vi "Invert Channel.vi"(8 "error in (no error)":errorcluster, 9 "Invert Channel (T: Enabled)":bool=TRUE, 10 "Channel (1: Channel 1)":u16(ring)=1 items=["Channel 1"=1, "Channel 2"=2, "Channel 3"=3, "Channel 4"=4], 11 "VISA resource name":refnum<visa-resource-name>) -> (0 "error out":errorcluster, 3 "VISA resource name out":refnum<visa-resource-name>)   [LabVIEW 2017, in "Tektronix TDS 200 1000 2000 Series.lvlib"]
doc: "Allows signals on all channels to be inverted."
uses:
  Tektronix TDS 200 1000 2000 Series.lvlib
panel:
  # "Enabled"
  # "Disabled"
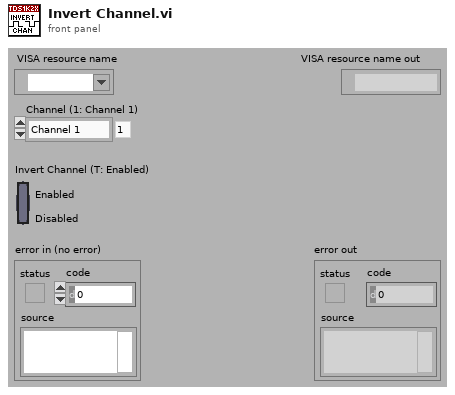
[diagram p1: front panel]
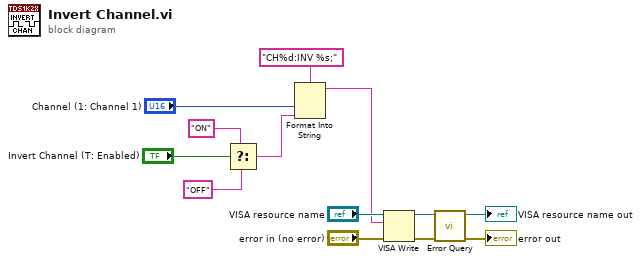
[diagram p0: block diagram]
diagram:
  n1 = Select(t="ON" ("multi-line string"), s="Invert Channel (T: Enabled)", f="OFF") -> (s? t:f=w1:string)
  n2 = Format Into String(format string="CH%d:INV %s;", "Channel (1: Channel 1)", w1) -> (resulting string=w5:string)  [unwired: 2 in, 1 out]
  n3 = VISA Write(VISA resource name="VISA resource name", write buffer=w5, error in (no error)="error in (no error)") -> (VISA resource name out=w10:refnum<visa-resource-name>, error out=w11:errorcluster)  [unwired: 1 out]
  n4 = call "Error Query.vi"("error in (no error)"=w11, "VISA resource name"=w10) -> ("error out"=→"error out":errorcluster, "VISA resource name out"=→"VISA resource name out":refnum<visa-resource-name>)  [unwired: 8 out]
